vi "Read File.vi"(8 "error in (no error)":errorcluster, 10 "Path in":path, 11 "File Interface in":refnum<class "File Interface.lvclass">) -> (0 "error out":errorcluster, 2 "SysDef":T1 {"Tree"."Properties"."Type" items=["K_STRING", "K_BOOL", "K_I32", "K_U32", "K_DOUBLE", "K_U64", "K_VARIANT", "K_DEPENDENTFILE", "K_DEPENDENTNODE", "K_DATASOURCENODE", "K_U16", "K_DBLARR", "K_U32ARR", "K_I32ARR", "K_STRINGARR", "K_DICTIONARY", "K_DICTIONARYARR"]})   [LabVIEW 2017, in "ImportExport.lvlib" / "File Interface.lvclass"]
uses:
  RefMem DMA Configuration.llb/File Interface.lvclass
  RefMem DMA Configuration.llb/SysDef.Export.ctl
  RefMem DMA Configuration.llb/TreeItem.ctl
  RefMem DMA Configuration.llb/TreeItem.Info.ctl
  RefMem DMA Configuration.llb/Custom Device Channel.ctl
  RefMem DMA Configuration.llb/Custom Device Channel Type.ctl
  RefMem DMA Configuration.llb/Custom Device Waveform.ctl
  RefMem DMA Configuration.llb/Custom Device Waveform DataType.ctl
  RefMem DMA Configuration.llb/TreeItem.Property.ctl
  RefMem DMA Configuration.llb/Advanced System Definition.lvlib
  RefMem DMA Configuration.llb/Custom Device API.lvlib
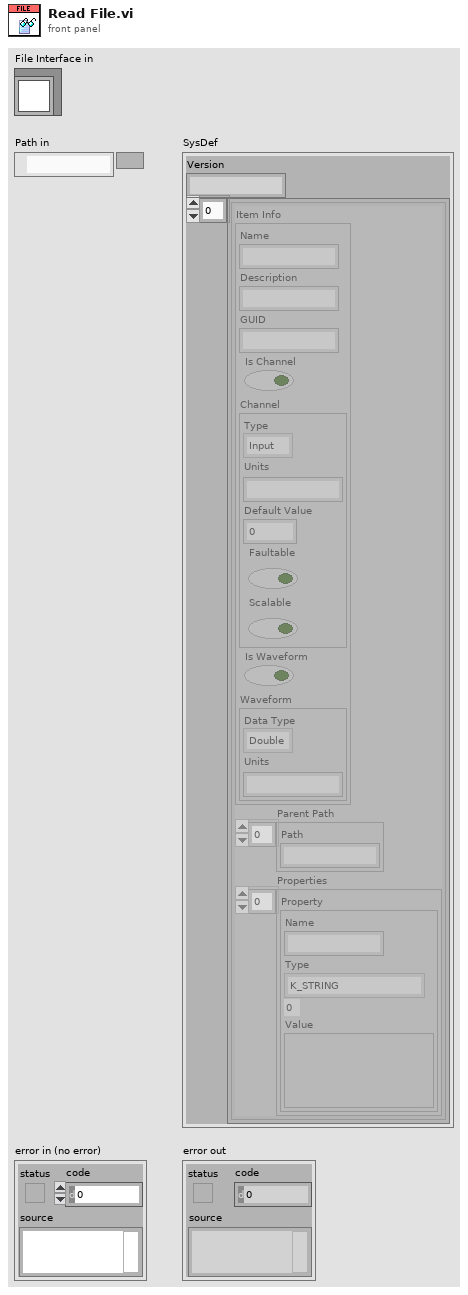
[diagram p1: front panel]
types:
  T1 = typedef "Advanced System Definition.lvlib/SysDef.Export.ctl" = cluster{"Version":string, "Tree":T2[]}
  T2 = typedef "Advanced System Definition.lvlib/TreeItem.ctl" = cluster{"Item Info":T3, "Parent Path":string[], "Properties":T8[]}
  T3 = typedef "Advanced System Definition.lvlib/TreeItem.Info.ctl" = cluster{"Name":string, "Description":string, "GUID":string, "Is Channel":bool, "Channel":T4, "Is Waveform":bool, "Waveform":T6}
  T4 = typedef "Custom Device API.lvlib/Custom Device Channel.ctl" = cluster{"Type":T5, "Units":string, "Default Value":dbl, "Faultable":bool, "Scalable":bool}
  T5 = typedef "Custom Device API.lvlib/Custom Device Channel Type.ctl" = enum16{"Input", "Output"}
  T6 = typedef "Custom Device API.lvlib/Custom Device Waveform.ctl" = cluster{"Data Type":T7, "Units":string}
  T7 = typedef "Custom Device API.lvlib/Custom Device Waveform DataType.ctl" = enum16{"Double", "Complex Double"}
  T8 = typedef "Advanced System Definition.lvlib/TreeItem.Property.ctl" = cluster{"Name":string, "Type":i32, "Value":variant}
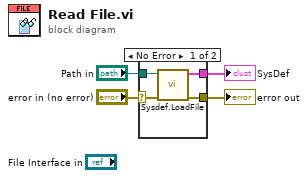
[diagram p0: block diagram]
diagram:
  n1 = case shown="No Error" "error in (no error)" {
    selector: "error in (no error)" -> [w6 w9]
    tunnel: [w5 w9] -> w3
    tunnel: "Path in" -> [w8 _]
    tunnel: [w7 _] -> w1
    frame No Error {
      n2 = call "Sysdef.LoadFile.vi"("error in (no error)"=w6, "Path in"=w8) -> ("error out"=w5:errorcluster, "SysDef"=w7:T1)  [unwired: 8 in]
    }
    frame Error {
    }
  }
  "error out" <- w3
  "SysDef" <- w1
